vi "Create.vi"(7 "File Type Interface Class (CSV)":refnum<class "File Type Interface.lvclass">) -> ()   [LabVIEW 2020, in "File Splitting Logger.lvclass"]
uses:
  File Splitting Logger.lvclass
  File Logger Interface/File Type Interface.lvclass
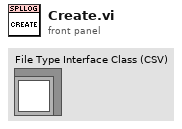
[diagram p1: front panel]
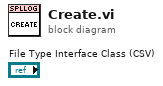
[diagram p0: block diagram]
diagram:
